vi "Advance_Slide_PP_SubVi.vi"(11 "Slide in":refnum<vi>) -> (3 "Slide":dbl(slide) scale=0.0..100.0)   [LabVIEW 2014]
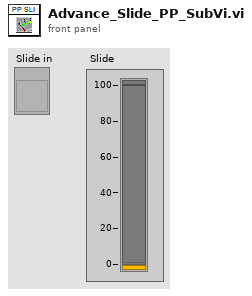
[diagram p1: front panel]
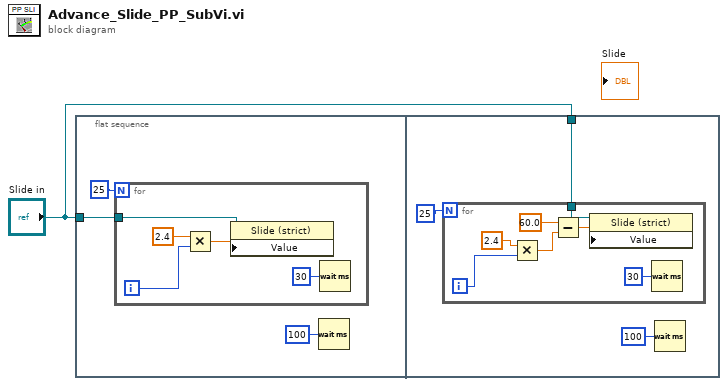
[diagram p0: block diagram]
diagram:
  n1 = flat-sequence {
    tunnel: "Slide in" -> [w2]
    tunnel: "Slide in" -> [w10]
    frame #0 {
      n2 = for {
        N: 25 -> [_]
        tunnel: w2 -> [w5]
        i -> [w7]
        n3 = Multiply(x=2.4, y=w7) -> (x*y=w6:dbl)
        n4 = property class="Slide (strict)"(reference=w5, "Value"=w6) -> ()  [unwired: 1 in, 2 out]
        n5 = Wait (ms)(milliseconds to wait=u32 30) -> ()  [unwired: 1 out]
      }
      n6 = Wait (ms)(milliseconds to wait=u32 100) -> ()  [unwired: 1 out]
    }
    frame #1 {
      n7 = for {
        N: 25 -> [_]
        tunnel: w10 -> [w13]
        i -> [w15]
        n8 = Multiply(x=2.4, y=w15) -> (x*y=w16:dbl)
        n9 = Subtract(x=60.0, y=w16) -> (x-y=w14:dbl)
        n10 = property class="Slide (strict)"(reference=w13, "Value"=w14) -> ()  [unwired: 1 in, 2 out]
        n11 = Wait (ms)(milliseconds to wait=u32 30) -> ()  [unwired: 1 out]
      }
      n12 = Wait (ms)(milliseconds to wait=u32 100) -> ()  [unwired: 1 out]
    }
  }
